vi "ts_M1M3SupportFPGA.vi"   [LabVIEW 2018]
uses:
  Common_FPGA_HealthAndStatus/DataTypes/HealthAndStatusSettings.ctl
  Common_FPGA_Modbus/DataTypes/ModbusPortSettings.ctl
  Common_FPGA_HealthAndStatus/DataTypes/HealthAndStatusFIFOCopySettings.ctl
  <vilib>/rvi/Emulation/niFpgaGetClockAttributes.vi
  <vilib>/rvi/Emulation/niFpgaSctlEmulationGetInTimedLoop.vi
  <vilib>/rvi/Emulation/niFpgaEmulationReportErrorSimple.vi
  <vilib>/rvi/eio/common/nirviEmuTemplateMethod_errors.vi
  <vilib>/rvi/Emulation/niFpgaCriticalErrorInLSC.vi
  <vilib>/eio/EIOMethodNode/EIOMethodNode.xnode
  Common_FPGA_HealthAndStatus/FPGAHealthAndStatus.lvlib
  Common_FPGA_Modbus/FPGAModbus.lvlib
types:
  T1 = typedef "FPGAHealthAndStatus.lvlib/HealthAndStatusFIFOCopySettings.ctl" = cluster{"InternalHealthAndStatusFIFO":refnum<k21>, "SourceHealthAndStatusFIFO":refnum<k21>}
  T2 = typedef "FPGAModbus.lvlib/ModbusPortSettings.ctl" = cluster{"TxPort":refnum<k21>, "TxDataFIFO":refnum<k21>, "TxInternalDataFIFO":refnum<k21>, "TxHealthAndStatusFIFO":refnum<k21>, "RxPort":refnum<k21>, "RxDataFIFO":refnum<k21>, "RxHealthAndStatusFIFO":refnum<k21>, "WaitForRxFrameRegister":refnum<k21>, "BaseHealthAndStatusAddress":u32, "IRQAddress":u8, "TriggerIRQRegister":refnum<k21>, "SoftwareControlledTrigger":refnum<k21>, "TimestampRegister":refnum<k21>, "TxTimestampFIFO":refnum<k21>}
  T3 = typedef "FPGAHealthAndStatus.lvlib/HealthAndStatusSettings.ctl" = cluster{"InternalHealthAndStatusFIFO":refnum<k21>, "HealthAndStatusQueryFIFO":refnum<k21>, "HealthAndStatusResponseFIFO":refnum<k21>, "HealthAndStatusMemory":refnum<k21>, "MemorySize":i32}
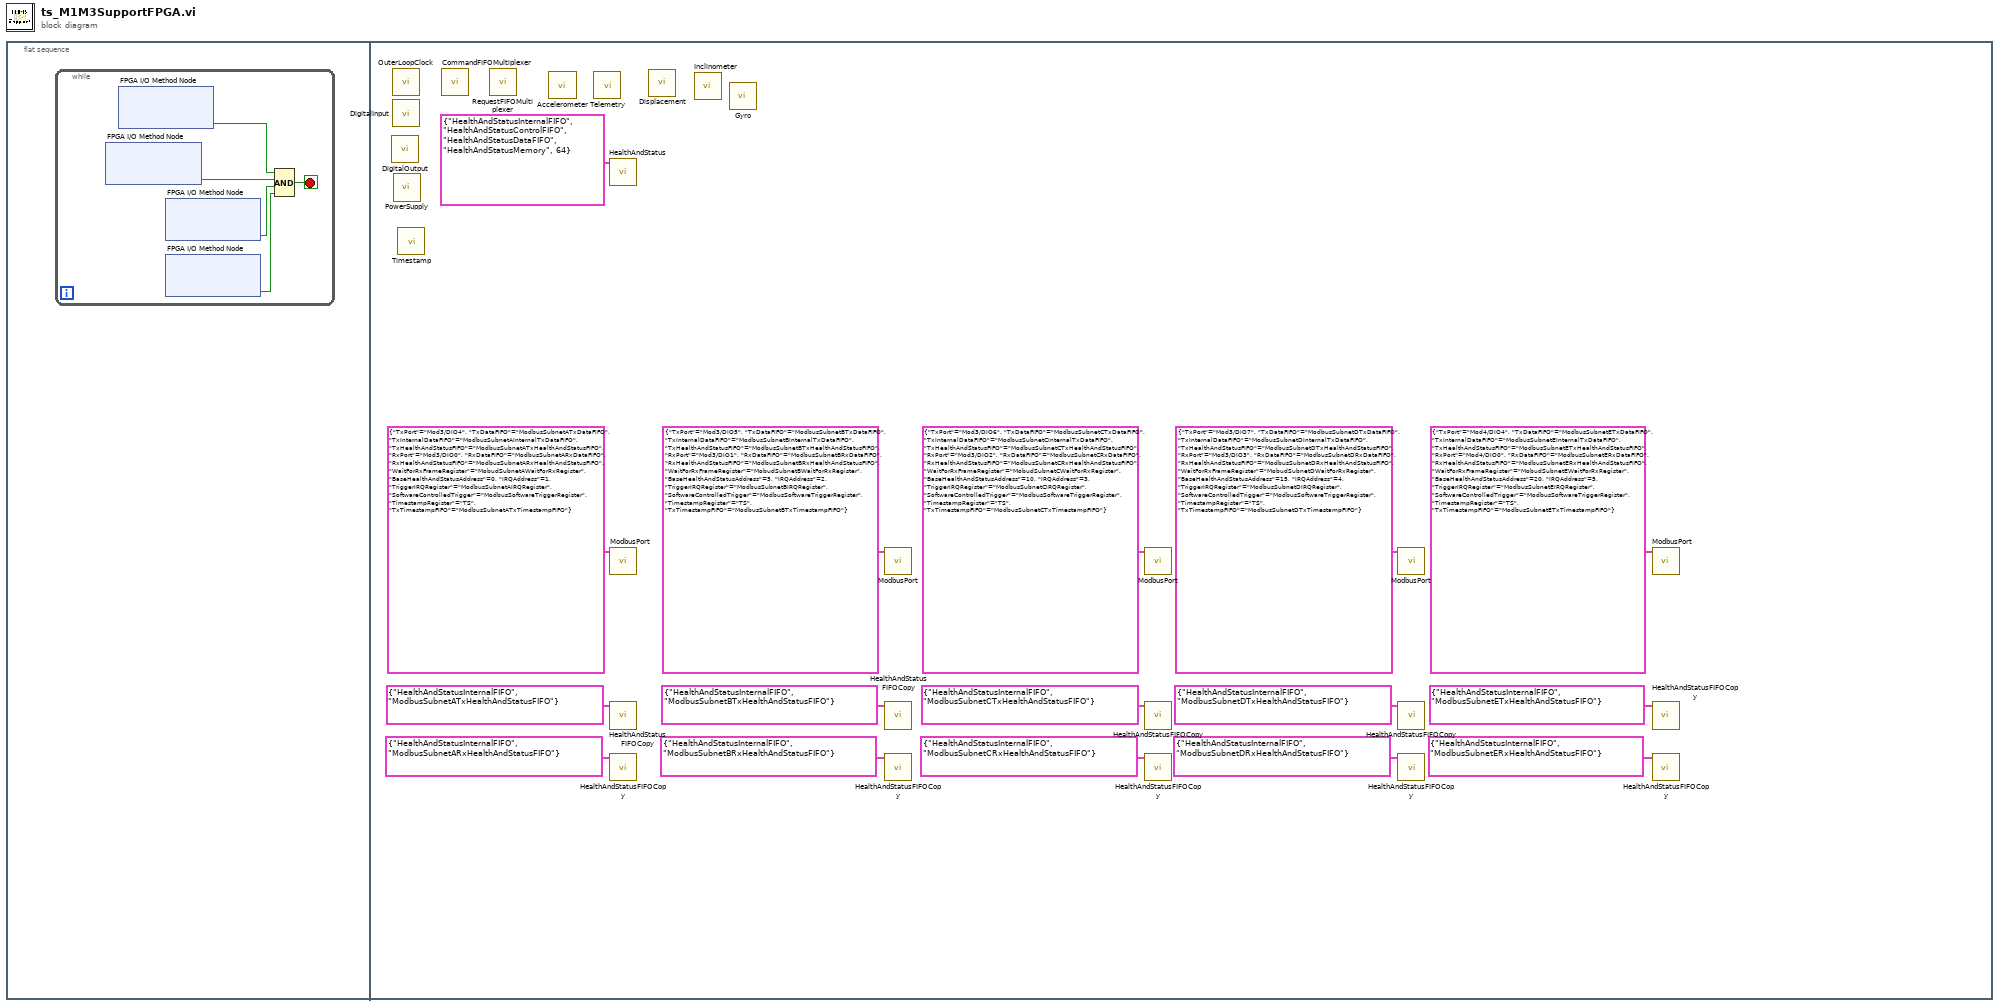
[diagram p0: block diagram]
diagram:
  n1 = flat-sequence {
    frame #0 {
      n2 = while {
        stop <- w1 stop-if-true
        n3 = xnode "FPGA I/O Method Node"() -> ("Ready"=w4:bool)  [unwired: 1 in, 1 out]
        n4 = xnode "FPGA I/O Method Node"() -> ("Ready"=w5:bool)  [unwired: 1 in, 1 out]
        n5 = xnode "FPGA I/O Method Node"() -> ("Ready"=w3:bool)  [unwired: 1 in, 1 out]
        n6 = xnode "FPGA I/O Method Node"() -> ("Ready"=w2:bool)  [unwired: 1 in, 1 out]
        n7 = Compound Arithmetic op=AND(w5, w4, w3, w2) -> (w1:bool)
      }
    }
    frame #1 {
      n8 = call "DigitalOutput.vi"() -> ()  [unwired: 12 in]
      n9 = call "OuterLoopClock.vi"() -> ()  [unwired: 12 in]
      n10 = call "DigitalInput.vi"() -> ()  [unwired: 12 in]
      n11 = call "PowerSupply.vi"() -> ()  [unwired: 12 in]
      n12 = call "Timestamp.vi"() -> ()  [unwired: 12 in]
      n13 = call "CommandFIFOMultiplexer.vi"() -> ()  [unwired: 12 in]
      n14 = call "RequestFIFOMultiplexer.vi"() -> ()  [unwired: 12 in]
      n15 = call "Accelerometer.vi"() -> ()  [unwired: 12 in]
      n16 = call "Telemetry.vi"() -> ()  [unwired: 12 in]
      n17 = call "HealthAndStatus.vi"("HealthAndStatusSettings"=T3 {"InternalHealthAndStatusFIFO"="HealthAndStatusInternalFIFO", "HealthAndStatusQueryFIFO"="HealthAndStatusControlFIFO", "HealthAndStatusResponseFIFO"="HealthAndStatusDataFIFO", "HealthAndStatusMemory"="HealthAndStatusMemory", "MemorySize"=64}) -> ()  [unwired: 11 in]
      n18 = call "ModbusPort.vi"("ModbusPortSettings"=T2 {"TxPort"="Mod3/DIO4", "TxDataFIFO"="ModbusSubnetATxDataFIFO", "TxInternalDataFIFO"="ModbusSubnetAInternalTxDataFIFO", "TxHealthAndStatusFIFO"="ModbusSubnetATxHealthAndStatusFIFO", "RxPort"="Mod3/DIO0", "RxDataFIFO"="ModbusSubnetARxDataFIFO", "RxHealthAndStatusFIFO"="ModbusSubnetARxHealthAndStatusFIFO", "WaitForRxFrameRegister"="MobudSubnetAWaitForRxRegister", "BaseHealthAndStatusAddress"=0, "IRQAddress"=1, "TriggerIRQRegister"="ModbusSubnetAIRQRegister", "SoftwareControlledTrigger"="ModbusSoftwareTriggerRegister", "TimestampRegister"="TS", "TxTimestampFIFO"="ModbusSubnetATxTimestampFIFO"}) -> ()  [unwired: 10 in]
      n19 = call "HealthAndStatusFIFOCopy.vi"("HealthAndStatusSettingsFIFOCopySettings"=T1 {"InternalHealthAndStatusFIFO"="HealthAndStatusInternalFIFO", "SourceHealthAndStatusFIFO"="ModbusSubnetATxHealthAndStatusFIFO"}) -> ()  [unwired: 11 in]
      n20 = call "HealthAndStatusFIFOCopy.vi"("HealthAndStatusSettingsFIFOCopySettings"=T1 {"InternalHealthAndStatusFIFO"="HealthAndStatusInternalFIFO", "SourceHealthAndStatusFIFO"="ModbusSubnetARxHealthAndStatusFIFO"}) -> ()  [unwired: 11 in]
      n21 = call "Displacement.vi"() -> ()  [unwired: 12 in]
      n22 = call "Inclinometer.vi"() -> ()  [unwired: 12 in]
      n23 = call "Gyro.vi"() -> ()  [unwired: 12 in]
      n24 = call "ModbusPort.vi"("ModbusPortSettings"=T2 {"TxPort"="Mod3/DIO5", "TxDataFIFO"="ModbusSubnetBTxDataFIFO", "TxInternalDataFIFO"="ModbusSubnetBInternalTxDataFIFO", "TxHealthAndStatusFIFO"="ModbusSubnetBTxHealthAndStatusFIFO", "RxPort"="Mod3/DIO1", "RxDataFIFO"="ModbusSubnetBRxDataFIFO", "RxHealthAndStatusFIFO"="ModbusSubnetBRxHealthAndStatusFIFO", "WaitForRxFrameRegister"="MobudSubnetBWaitForRxRegister", "BaseHealthAndStatusAddress"=5, "IRQAddress"=2, "TriggerIRQRegister"="ModbusSubnetBIRQRegister", "SoftwareControlledTrigger"="ModbusSoftwareTriggerRegister", "TimestampRegister"="TS", "TxTimestampFIFO"="ModbusSubnetBTxTimestampFIFO"}) -> ()  [unwired: 10 in]
      n25 = call "HealthAndStatusFIFOCopy.vi"("HealthAndStatusSettingsFIFOCopySettings"=T1 {"InternalHealthAndStatusFIFO"="HealthAndStatusInternalFIFO", "SourceHealthAndStatusFIFO"="ModbusSubnetBTxHealthAndStatusFIFO"}) -> ()  [unwired: 11 in]
      n26 = call "HealthAndStatusFIFOCopy.vi"("HealthAndStatusSettingsFIFOCopySettings"=T1 {"InternalHealthAndStatusFIFO"="HealthAndStatusInternalFIFO", "SourceHealthAndStatusFIFO"="ModbusSubnetBRxHealthAndStatusFIFO"}) -> ()  [unwired: 11 in]
      n27 = call "ModbusPort.vi"("ModbusPortSettings"=T2 {"TxPort"="Mod3/DIO6", "TxDataFIFO"="ModbusSubnetCTxDataFIFO", "TxInternalDataFIFO"="ModbusSubnetCInternalTxDataFIFO", "TxHealthAndStatusFIFO"="ModbusSubnetCTxHealthAndStatusFIFO", "RxPort"="Mod3/DIO2", "RxDataFIFO"="ModbusSubnetCRxDataFIFO", "RxHealthAndStatusFIFO"="ModbusSubnetCRxHealthAndStatusFIFO", "WaitForRxFrameRegister"="MobudSubnetCWaitForRxRegister", "BaseHealthAndStatusAddress"=10, "IRQAddress"=3, "TriggerIRQRegister"="ModbusSubnetCIRQRegister", "SoftwareControlledTrigger"="ModbusSoftwareTriggerRegister", "TimestampRegister"="TS", "TxTimestampFIFO"="ModbusSubnetCTxTimestampFIFO"}) -> ()  [unwired: 10 in]
      n28 = call "HealthAndStatusFIFOCopy.vi"("HealthAndStatusSettingsFIFOCopySettings"=T1 {"InternalHealthAndStatusFIFO"="HealthAndStatusInternalFIFO", "SourceHealthAndStatusFIFO"="ModbusSubnetCTxHealthAndStatusFIFO"}) -> ()  [unwired: 11 in]
      n29 = call "HealthAndStatusFIFOCopy.vi"("HealthAndStatusSettingsFIFOCopySettings"=T1 {"InternalHealthAndStatusFIFO"="HealthAndStatusInternalFIFO", "SourceHealthAndStatusFIFO"="ModbusSubnetCRxHealthAndStatusFIFO"}) -> ()  [unwired: 11 in]
      n30 = call "ModbusPort.vi"("ModbusPortSettings"=T2 {"TxPort"="Mod3/DIO7", "TxDataFIFO"="ModbusSubnetDTxDataFIFO", "TxInternalDataFIFO"="ModbusSubnetDInternalTxDataFIFO", "TxHealthAndStatusFIFO"="ModbusSubnetDTxHealthAndStatusFIFO", "RxPort"="Mod3/DIO3", "RxDataFIFO"="ModbusSubnetDRxDataFIFO", "RxHealthAndStatusFIFO"="ModbusSubnetDRxHealthAndStatusFIFO", "WaitForRxFrameRegister"="MobudSubnetDWaitForRxRegister", "BaseHealthAndStatusAddress"=15, "IRQAddress"=4, "TriggerIRQRegister"="ModbusSubnetDIRQRegister", "SoftwareControlledTrigger"="ModbusSoftwareTriggerRegister", "TimestampRegister"="TS", "TxTimestampFIFO"="ModbusSubnetDTxTimestampFIFO"}) -> ()  [unwired: 10 in]
      n31 = call "HealthAndStatusFIFOCopy.vi"("HealthAndStatusSettingsFIFOCopySettings"=T1 {"InternalHealthAndStatusFIFO"="HealthAndStatusInternalFIFO", "SourceHealthAndStatusFIFO"="ModbusSubnetDTxHealthAndStatusFIFO"}) -> ()  [unwired: 11 in]
      n32 = call "HealthAndStatusFIFOCopy.vi"("HealthAndStatusSettingsFIFOCopySettings"=T1 {"InternalHealthAndStatusFIFO"="HealthAndStatusInternalFIFO", "SourceHealthAndStatusFIFO"="ModbusSubnetDRxHealthAndStatusFIFO"}) -> ()  [unwired: 11 in]
      n33 = call "ModbusPort.vi"("ModbusPortSettings"=T2 {"TxPort"="Mod4/DIO4", "TxDataFIFO"="ModbusSubnetETxDataFIFO", "TxInternalDataFIFO"="ModbusSubnetEInternalTxDataFIFO", "TxHealthAndStatusFIFO"="ModbusSubnetETxHealthAndStatusFIFO", "RxPort"="Mod4/DIO0", "RxDataFIFO"="ModbusSubnetERxDataFIFO", "RxHealthAndStatusFIFO"="ModbusSubnetERxHealthAndStatusFIFO", "WaitForRxFrameRegister"="MobudSubnetEWaitForRxRegister", "BaseHealthAndStatusAddress"=20, "IRQAddress"=5, "TriggerIRQRegister"="ModbusSubnetEIRQRegister", "SoftwareControlledTrigger"="ModbusSoftwareTriggerRegister", "TimestampRegister"="TS", "TxTimestampFIFO"="ModbusSubnetETxTimestampFIFO"}) -> ()  [unwired: 10 in]
      n34 = call "HealthAndStatusFIFOCopy.vi"("HealthAndStatusSettingsFIFOCopySettings"=T1 {"InternalHealthAndStatusFIFO"="HealthAndStatusInternalFIFO", "SourceHealthAndStatusFIFO"="ModbusSubnetETxHealthAndStatusFIFO"}) -> ()  [unwired: 11 in]
      n35 = call "HealthAndStatusFIFOCopy.vi"("HealthAndStatusSettingsFIFOCopySettings"=T1 {"InternalHealthAndStatusFIFO"="HealthAndStatusInternalFIFO", "SourceHealthAndStatusFIFO"="ModbusSubnetERxHealthAndStatusFIFO"}) -> ()  [unwired: 11 in]
    }
  }
